vi "Initialize Instrument.vi"(8 "error in (no error)":errorcluster, 10 "Reset":bool, 11 "VNA-CMT S2 S4 in":refnum<class "VNA-CMT S2 S4.lvclass">) -> (0 "error out":errorcluster, 3 "VNA-CMT S2 S4 out":refnum<class "VNA-CMT S2 S4.lvclass">)   [LabVIEW 2020, in "VNA-CMT S2 S4.lvclass"]
uses:
  VNA-CMT S2 S4.lvclass
  C:/Sandbox/RF Bench/Source Code/WiSpry Test Framework/Instruments/Instrument.lvclass
  C:/Sandbox/RF Bench/Source Code/WiSpry Test Framework/Instruments/Vector Network Analyzer/Vector Network Analyzer.lvclass
  Instrument.lvclass/Instrument.ctl
  Vector Network Analyzer.lvclass/Vector Network Analyzer.ctl
  Instrument.lvclass
  Vector Network Analyzer.lvclass
  <instrlib>/Keysight PNA Series/Keysight PNA Series.lvlib
  <instrlib>/CMT S2 and S4 VNA/CMT S2 and S4 VNA.lvlib
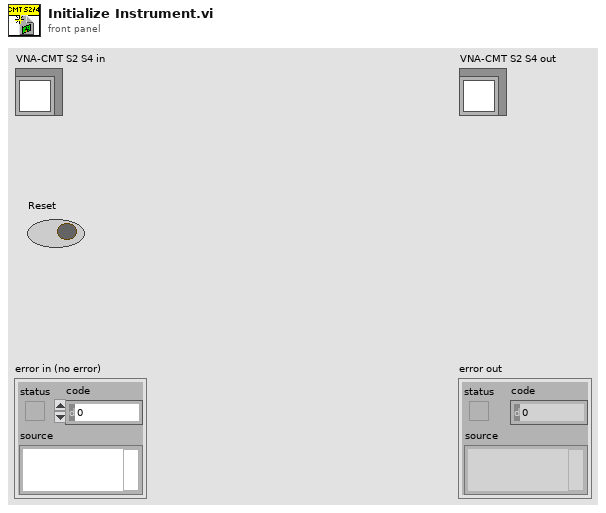
[diagram p1: front panel]
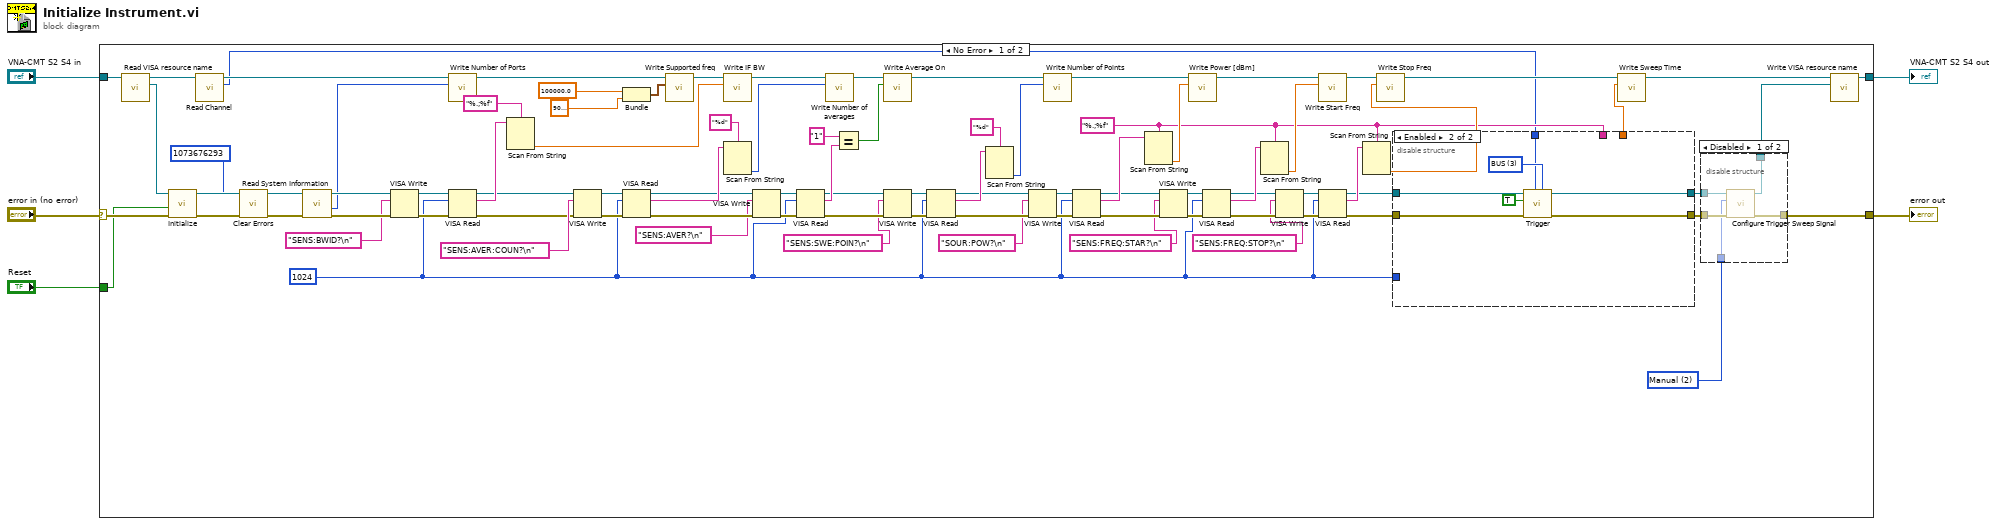
[diagram p0: block diagram]
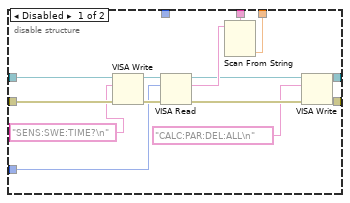
[diagram p2: hidden frame]
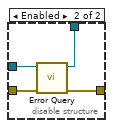
[diagram p3: hidden frame]
diagram:
  n1 = case shown="No Error" "error in (no error)" {
    selector: "error in (no error)" -> [w30 w125]
    tunnel: "VNA-CMT S2 S4 in" -> [w31 w126]
    tunnel: [w34 w125] -> w5
    tunnel: [w78 w126] -> w4
    tunnel: "Reset" -> [w28 _]
    frame No Error {
      w32 = 2 items=["Immediate", "External", "Manual"] ("Trigger Source (0: Immediate)")
      w38 = "%.;%f" ("format string")
      w14 = u32 1024 ("byte count")
      n2 = call "Read VISA resource name.vi"("Instrument in"=w31) -> ("VISA resource name"=w29:refnum<visa-resource-name>, "Instrument out"=w7:refnum<class "VNA-CMT S2 S4.lvclass">)  [unwired: 9 in]
      n3 = call <instrlib>:"Initialize.vi"("error in (no error)"=w30, "Reset? (T: Yes)"=w28, "VISA resource name"=w29) -> ("error out"=w22:errorcluster, "VISA resource name out"=w27:refnum<visa-resource-name>)  [unwired: 6 in, 1 out]
      n4 = call-dynamic "Read Channel.vi"("Vector Network Analyzer in"=w7) -> ("Channel"=w6:i32, "Vector Network Analyzer out"=w8:refnum<class "VNA-CMT S2 S4.lvclass">)  [unwired: 9 in]
      n5 = call <vilib>:"Clear Errors.vi"("error in (no error)"=w22, "specific error code to clear (0: all)"=1073676293) -> ("error out"=w20:errorcluster)  [unwired: 4 in, 1 out]
      n6 = call <instrlib>:"Read System Information.vi"("error in (no error)"=w20, "VISA resource name"=w27) -> ("error out"=w25:errorcluster, "Number of Ports"=w24:i32, "VISA resource name out"=w26:refnum<visa-resource-name>)  [unwired: 5 in, 2 out]
      n7 = VISA Write(VISA resource name=w26, write buffer="SENS:BWID?\n", error in (no error)=w25) -> (VISA resource name out=w84:refnum<visa-resource-name>, error out=w83:errorcluster)  [unwired: 1 out]
      n8 = call "Write Number of Ports.vi"("Number of Ports"=w24, "Vector Network Analyzer in"=w8) -> ("Vector Network Analyzer out"=w94:refnum<class "VNA-CMT S2 S4.lvclass">)  [unwired: 9 in]
      n9 = VISA Read(VISA resource name=w84, byte count=w14, error in (no error)=w83) -> (VISA resource name out=w18:refnum<visa-resource-name>, read buffer=w81:string, error out=w17:errorcluster)  [unwired: 1 out]
      n10 = Scan From String(format string="%.;%f", input string=w81) -> (output 1=w80:dbl)  [unwired: 3 in, 3 out]
      n11 = VISA Write(VISA resource name=w18, write buffer="SENS:AVER:COUN?\n", error in (no error)=w17) -> (VISA resource name out=w16:refnum<visa-resource-name>, error out=w15:errorcluster)  [unwired: 1 out]
      n12 = Bundle(100000.0, 9000000000.0) -> (w93:cluster{dbl, dbl})  [unwired: 1 in]
      n13 = VISA Read(VISA resource name=w16, byte count=w14, error in (no error)=w15) -> (VISA resource name out=w72:refnum<visa-resource-name>, read buffer=w77:string, error out=w71:errorcluster)  [unwired: 1 out]
      n14 = call "Write Supported freq.vi"("Supported freq"=w93, "Vector Network Analyzer in"=w94) -> ("Vector Network Analyzer out"=w79:refnum<class "VNA-CMT S2 S4.lvclass">)  [unwired: 9 in]
      n15 = call "Write IF BW.vi"("IF BW"=w80, "Vector Network Analyzer in"=w79) -> ("Vector Network Analyzer out"=w92:refnum<class "VNA-CMT S2 S4.lvclass">)  [unwired: 9 in]
      n16 = Scan From String(format string="%d", input string=w77) -> (output 1=w75:i32)  [unwired: 3 in, 3 out]
      n17 = VISA Write(VISA resource name=w72, write buffer="SENS:AVER?\n", error in (no error)=w71) -> (VISA resource name out=w74:refnum<visa-resource-name>, error out=w73:errorcluster)  [unwired: 1 out]
      n18 = VISA Read(VISA resource name=w74, byte count=w14, error in (no error)=w73) -> (VISA resource name out=w65:refnum<visa-resource-name>, read buffer=w70:string, error out=w64:errorcluster)  [unwired: 1 out]
      n19 = call "Write Number of averages.vi"("Number of averages"=w75, "Vector Network Analyzer in"=w92) -> ("Vector Network Analyzer out"=w91:refnum<class "VNA-CMT S2 S4.lvclass">)  [unwired: 9 in]
      n20 = Equal?(x="1", y=w70) -> (x = y?=w68:bool)
      n21 = call "Write Average On.vi"("Average On"=w68, "Vector Network Analyzer in"=w91) -> ("Vector Network Analyzer out"=w90:refnum<class "VNA-CMT S2 S4.lvclass">)  [unwired: 9 in]
      n22 = VISA Write(VISA resource name=w65, write buffer="SENS:SWE:POIN?\n", error in (no error)=w64) -> (VISA resource name out=w66:refnum<visa-resource-name>, error out=w67:errorcluster)  [unwired: 1 out]
      n23 = VISA Read(VISA resource name=w66, byte count=w14, error in (no error)=w67) -> (VISA resource name out=w58:refnum<visa-resource-name>, read buffer=w62:string, error out=w57:errorcluster)  [unwired: 1 out]
      n24 = Scan From String(format string="%d", input string=w62) -> (output 1=w61:i32)  [unwired: 3 in, 3 out]
      n25 = VISA Write(VISA resource name=w58, write buffer="SOUR:POW?\n", error in (no error)=w57) -> (VISA resource name out=w60:refnum<visa-resource-name>, error out=w59:errorcluster)  [unwired: 1 out]
      n26 = call "Write Number of Points.vi"("Number of Points"=w61, "Vector Network Analyzer in"=w90) -> ("Vector Network Analyzer out"=w89:refnum<class "VNA-CMT S2 S4.lvclass">)  [unwired: 9 in]
      n27 = VISA Read(VISA resource name=w60, byte count=w14, error in (no error)=w59) -> (VISA resource name out=w52:refnum<visa-resource-name>, read buffer=w56:string, error out=w51:errorcluster)  [unwired: 1 out]
      n28 = Scan From String(format string=w38, input string=w56) -> (output 1=w55:dbl)  [unwired: 3 in, 3 out]
      n29 = VISA Write(VISA resource name=w52, write buffer="SENS:FREQ:STAR?\n", error in (no error)=w51) -> (VISA resource name out=w53:refnum<visa-resource-name>, error out=w54:errorcluster)  [unwired: 1 out]
      n30 = call "Write Power [dBm].vi"("Power [dBm]"=w55, "Vector Network Analyzer in"=w89) -> ("Vector Network Analyzer out"=w88:refnum<class "VNA-CMT S2 S4.lvclass">)  [unwired: 9 in]
      n31 = VISA Read(VISA resource name=w53, byte count=w14, error in (no error)=w54) -> (VISA resource name out=w47:refnum<visa-resource-name>, read buffer=w50:string, error out=w46:errorcluster)  [unwired: 1 out]
      n32 = Scan From String(format string=w38, input string=w50) -> (output 1=w49:dbl)  [unwired: 3 in, 3 out]
      n33 = VISA Write(VISA resource name=w47, write buffer="SENS:FREQ:STOP?\n", error in (no error)=w46) -> (VISA resource name out=w48:refnum<visa-resource-name>, error out=w45:errorcluster)  [unwired: 1 out]
      n34 = call "Write Start Freq.vi"("Start Freq"=w49, "Vector Network Analyzer in"=w88) -> ("Vector Network Analyzer out"=w87:refnum<class "VNA-CMT S2 S4.lvclass">)  [unwired: 9 in]
      n35 = VISA Read(VISA resource name=w48, byte count=w14, error in (no error)=w45) -> (VISA resource name out=w42:refnum<visa-resource-name>, read buffer=w43:string, error out=w41:errorcluster)  [unwired: 1 out]
      n36 = Scan From String(format string=w38, input string=w43) -> (output 1=w44:dbl)  [unwired: 3 in, 3 out]
      n37 = call "Write Stop Freq.vi"("Stop Freq"=w44, "Vector Network Analyzer in"=w87) -> ("Vector Network Analyzer out"=w40:refnum<class "VNA-CMT S2 S4.lvclass">)  [unwired: 9 in]
      n38 = disable-structure shown="Enabled" {
        disable-tunnel: w42 -> [w106 w114]
        disable-tunnel: w41 -> [w105 w115]
        disable-tunnel: w38 -> [w103 _]
        disable-tunnel: [w102 _] -> w37
        disable-tunnel: [w99 w112] -> w36
        disable-tunnel: [w98 w113] -> w35
        disable-tunnel: w14 -> [w97 _]
        disable-tunnel: w6 -> [_ w109]
        frame Disabled {
          n39 = VISA Write(VISA resource name=w106, write buffer="SENS:SWE:TIME?\n", error in (no error)=w105) -> (VISA resource name out=w107:refnum<visa-resource-name>, error out=w108:errorcluster)  [unwired: 1 out]
          n40 = VISA Read(VISA resource name=w107, byte count=w97, error in (no error)=w108) -> (VISA resource name out=w100:refnum<visa-resource-name>, read buffer=w104:string, error out=w101:errorcluster)  [unwired: 1 out]
          n41 = Scan From String(format string=w103, input string=w104) -> (output 1=w102:dbl)  [unwired: 3 in, 3 out]
          n42 = VISA Write(VISA resource name=w100, write buffer="CALC:PAR:DEL:ALL\n", error in (no error)=w101) -> (VISA resource name out=w99:refnum<visa-resource-name>, error out=w98:errorcluster)  [unwired: 1 out]
        }
        frame Enabled {
          w111 = u16 3 items=["Internal", "External", "Manual", "BUS"] ("Trigger Source (0: Internal)")
          n43 = call <instrlib>:"Trigger.vi"("Trigger Source (0: Internal)"=w111, "Channel (1)"=w109, "error in (no error)"=w115, "Continuous Sweep (T: Enable)"=TRUE, "VISA resource name"=w114) -> ("error out"=w113:errorcluster, "VISA resource name out"=w112:refnum<visa-resource-name>)  [unwired: 5 in]
        }
      }
      n44 = call "Write Sweep Time.vi"("Sweep Time"=w37, "Vector Network Analyzer in"=w40) -> ("Vector Network Analyzer out"=w39:refnum<class "VNA-CMT S2 S4.lvclass">)  [unwired: 9 in]
      n45 = disable-structure shown="Disabled" {
        disable-tunnel: w36 -> [w120 w123]
        disable-tunnel: w35 -> [w119 w124]
        disable-tunnel: [w118 w122] -> w34
        disable-tunnel: [w117 w121] -> w33
        disable-tunnel: w32 -> [w116 _]
        frame Disabled {
          n46 = call <instrlib>:"Configure Trigger Sweep Signal.vi"("error in (no error)"=w119, "Trigger Source (0: Immediate)"=w116, "VISA resource name"=w120) -> ("error out"=w118:errorcluster, "VISA resource name out"=w117:refnum<visa-resource-name>)  [unwired: 7 in]
        }
        frame Enabled {
          n47 = call <instrlib>:"Error Query.vi"("error in (no error)"=w124, "VISA resource name"=w123) -> ("error out"=w122:errorcluster, "VISA resource name out"=w121:refnum<visa-resource-name>)  [unwired: 6 in, 2 out]
        }
      }
      n48 = call "Write VISA resource name.vi"("VISA resource name"=w33, "Instrument in"=w39) -> ("Instrument out"=w78:refnum<class "VNA-CMT S2 S4.lvclass">)  [unwired: 9 in]
    }
    frame Error {
    }
  }
  "error out" <- w5
  "VNA-CMT S2 S4 out" <- w4
